vi "initialize.vi"(0 "HB_Simple":refnum<class "HB_Simple.lvclass">, 3 "initializationData":variant, 5 "error in (no error)":errorcluster, 7 "binaryString":string, 8 "I8 Array":i8[](array[numeric]), 9 "prependSize? (T)":bool, 11 "byteOrder (0:big-endian, network order)":T1(ring)) -> (14 "dup HB_Simple":refnum<class "HB_Simple.lvclass">, 17 "found?":bool, 19 "error out":errorcluster)   [LabVIEW 2009, in "HB_BaseClass_Examples.lvlib" / "HB_Simple.lvclass"]
doc: "This is a dynamic dispatch VI to be implemented by child classes to initialize their attributes.\n\n<B>Recommendation:</B> Use Variant for initialization data."
uses:
  HB_Simple.lvclass
  lib.lib/HGF_LVC/HGF_BaseClasses/HGF_TriggeredEvent/HGF_TriggeredEvent.lvclass
  lib.lib/HGF_LVC/HGF_BaseClasses/HGF_PVPublisher/HGF_PVPublisher.lvclass
  lib.lib/HGF_LVC/HGF_BaseClasses/HGF_Visitable/HGF_Visitable.lvclass
  HB_Simple.lvclass/HB_Simple.ctl
  lib.lib/HGF_LVC/HGF_BaseClasses/HGF_Factory/HGF_Factory.lvclass
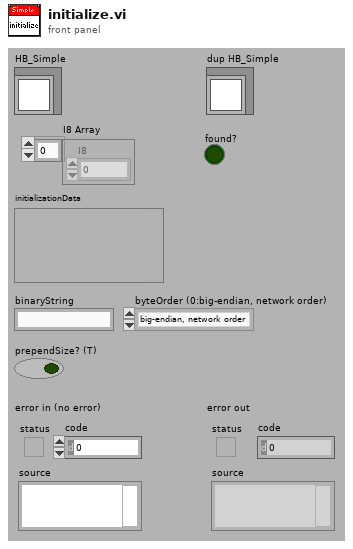
[diagram p1: front panel]
types:
  T1 = enum16{"big-endian, network order", "native, host order", "little-endian"}
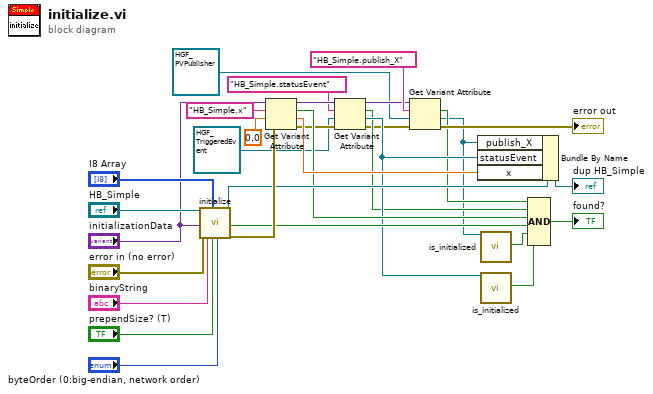
[diagram p0: block diagram]
diagram:
  n1 = call-parent "initialize.vi"("HGF_Base"="HB_Simple", "initializationData"="initializationData", "error in (no error)"="error in (no error)", "binaryString"="binaryString", "I8 Array"="I8 Array", "prependSize? (T)"="prependSize? (T)", "byteOrder (0:big-endian, network order)"="byteOrder (0:big-endian, network order)") -> ("dup HGF_Base"=w23:refnum<class "HB_Simple.lvclass">, "found?"=w19:bool, "error out"=w27:errorcluster)  [unwired: 1 in, 9 out]
  n2 = Get Variant Attribute(Variant="initializationData", name="HB_Simple.x", default value (empty Variant)=0.0, error in=w27) -> (duplicate Variant=w13:variant, found=w20:bool, value=w21:dbl, error out=w14:errorcluster)
  n3 = Get Variant Attribute(Variant=w13, name="HB_Simple.statusEvent", default value (empty Variant)=refnum<class "HGF_TriggeredEvent.lvclass"> refnum ("statusEvent"), error in=w14) -> (duplicate Variant=w5:variant, found=w10:bool, value=w11:refnum<class "HGF_TriggeredEvent.lvclass">, error out=→"error out":errorcluster)
  n4 = Get Variant Attribute(Variant=w5, name="HB_Simple.publish_X", default value (empty Variant)=refnum<class "HGF_PVPublisher.lvclass"> refnum ("publish_X")) -> (found=w4:bool, value=w2:refnum<class "HGF_PVPublisher.lvclass">)  [unwired: 1 in, 2 out]
  n5 = Bundle By Name(cluster=w23, "publish_X"=w2, "statusEvent"=w11, "x"=w21) -> (→"dup HB_Simple":refnum<class "HB_Simple.lvclass">)
  n6 = call "is_initialized.vi"("HGF_Factory"=w2) -> ("initialized?"=w1:bool)  [unwired: 1 in, 17 out]
  n7 = call "is_initialized.vi"("HGF_Factory"=w11) -> ("initialized?"=w9:bool)  [unwired: 1 in, 17 out]
  n8 = Compound Arithmetic op=AND(w4, w10, w20, w19, w1, w9) -> (→"found?":bool)
